vi "Scale Line Segment.vi"(8 "error in":errorcluster, 9 "Scale Factor":dbl=1.0, 10 "Point B in":refnum<class "Vec3d Class.lvclass">, 11 "Point A in":refnum<class "Vec3d Class.lvclass">) -> (0 "error out":errorcluster, 2 "Point B out":refnum<class "Vec3d Class.lvclass">, 3 "Point A out":refnum<class "Vec3d Class.lvclass">)   [LabVIEW 2017]
uses:
  Vec3d Class/Vec3d Class.lvclass
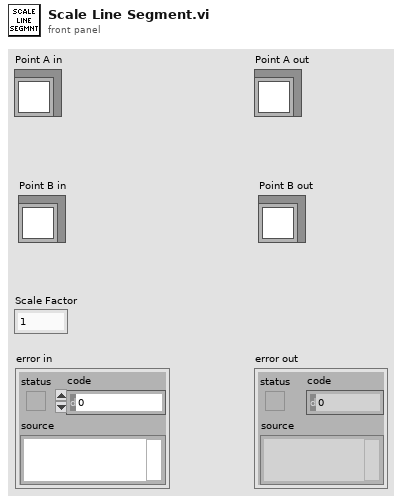
[diagram p1: front panel]
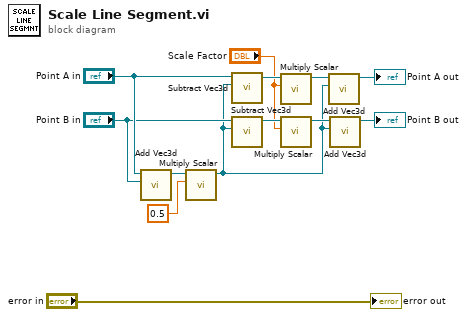
[diagram p0: block diagram]
diagram:
  n1 = call-dynamic "Add Vec3d.vi"(10:"Vec3d Class in"="Point B in", 11:"Vec3d Class in"="Point A in") -> ("Vec3d Class out"=w13:refnum<class "Vec3d Class.lvclass">)  [unwired: 8 in, 1 out]
  n2 = call-dynamic "Multiply Scalar.vi"("Scale"=0.5, "Vec3d in"=w13) -> ("Vec3d out"=w4:refnum<class "Vec3d Class.lvclass">)  [unwired: 8 in, 1 out]
  n3 = call "Subtract Vec3d.vi"("Vec3d in 2"=w4, "Vec3d in 1"="Point A in") -> ("Vec3d Class out"=w9:refnum<class "Vec3d Class.lvclass">)  [unwired: 8 in, 1 out]
  n4 = call "Subtract Vec3d.vi"("Vec3d in 2"=w4, "Vec3d in 1"="Point B in") -> ("Vec3d Class out"=w8:refnum<class "Vec3d Class.lvclass">)  [unwired: 8 in, 1 out]
  n5 = call-dynamic "Multiply Scalar.vi"("Scale"="Scale Factor", "Vec3d in"=w9) -> ("Vec3d out"=w6:refnum<class "Vec3d Class.lvclass">)  [unwired: 8 in, 1 out]
  n6 = call-dynamic "Multiply Scalar.vi"("Scale"="Scale Factor", "Vec3d in"=w8) -> ("Vec3d out"=w5:refnum<class "Vec3d Class.lvclass">)  [unwired: 8 in, 1 out]
  n7 = call-dynamic "Add Vec3d.vi"(10:"Vec3d Class in"=w4, 11:"Vec3d Class in"=w6) -> ("Vec3d Class out"=→"Point A out":refnum<class "Vec3d Class.lvclass">)  [unwired: 8 in, 1 out]
  n8 = call-dynamic "Add Vec3d.vi"(10:"Vec3d Class in"=w4, 11:"Vec3d Class in"=w5) -> ("Vec3d Class out"=→"Point B out":refnum<class "Vec3d Class.lvclass">)  [unwired: 8 in, 1 out]
  "error out" <- "error in"
